vi "LearningVI_4_LongAvg.vi"() -> ()   [LabVIEW 2013]
uses:
  <vilib>/Analysis/baseanly.llb/Mean (DBL).vi
  <vilib>/Analysis/NI_AALBase.lvlib
panel:
  out "DC Value":dbl[](array[numeric]) format="%#.6f"
  in  "How many samples\nto average?":dbl
  in  "Saving Avg?":bool
  in  "Filename":path=path "trial_1.lvm"
  out "Samples Indicator":dbl
  in  "STOP":bool
  in  "Save Waveform":bool
  out "Peak2Peak V":dbl[](array[numeric])
  out "Waveform Chart":dynamicdata(graph)
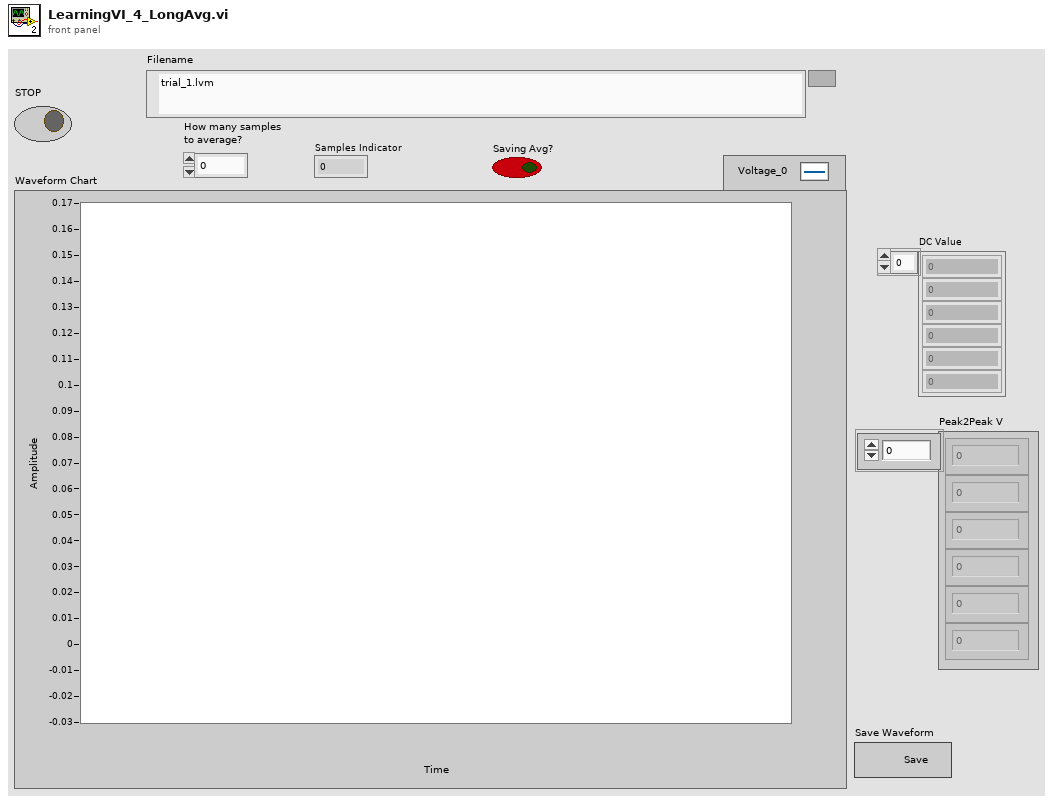
[diagram p1: front panel]
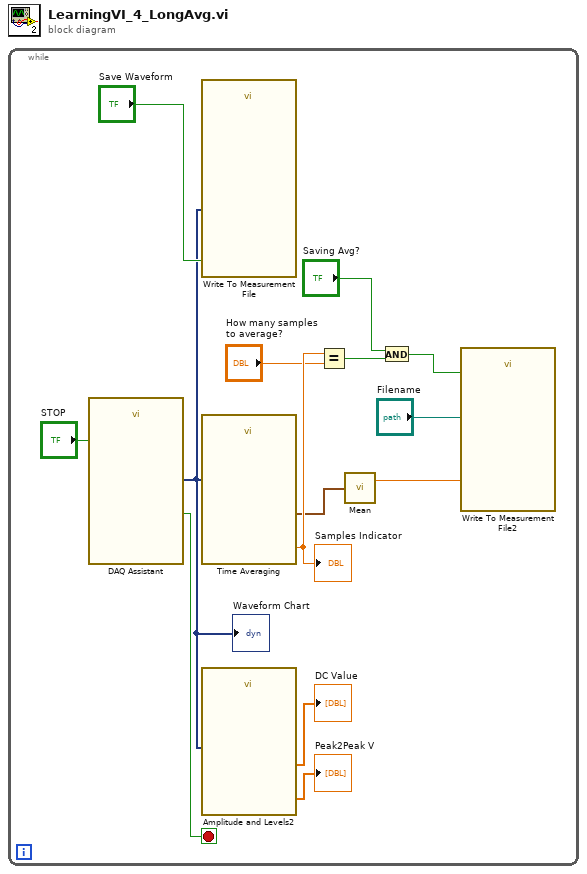
[diagram p0: block diagram]
diagram:
  n1 = while {
    stop <- w14 stop-if-true
    n2 = call "DAQ Assistant"("stop (F)"="STOP") -> ("data"=w4:dynamicdata, "stopped"=w14:bool)  [unwired: 15 in, 2 out]
    "Waveform Chart" <- w4
    n3 = call "Write To Measurement File"("Signals"=w4, "Enable"="Save Waveform") -> ()  [unwired: 15 in, 3 out]
    n4 = call "Time Averaging"("input signal"=w4) -> ("time avg. signal"=w2:waveform(dbl), "avg. counter"=w10:dbl)  [unwired: 15 in, 2 out]
    "Samples Indicator" <- w10
    n5 = call "Amplitude and Levels2"("input signals"=w4) -> ("dc"=→"DC Value":dbl[], "peak-peak"=→"Peak2Peak V":dbl[])  [unwired: 15 in, 2 out]
    n6 = Equal?(x=w10, y="How many samples\nto average?") -> (x = y?=w7:bool)
    n7 = call-poly <vilib>:"Mean.vi"("X"=w2) -> ("mean"=w1:dbl)  [unwired: 1 out]
    n8 = And(x="Saving Avg?", y=w7) -> (x .and. y?=w6:bool)
    n9 = call "Write To Measurement File2"("Signals"=w1, "Enable"=w6, "Filename"="Filename") -> ()  [unwired: 14 in, 3 out]
  }
